vi "Drive Distance to Turn Angle.vi"(5 "Wheelbase (in)":dbl=21.5, 9 "Distance (in)":dbl) -> (3 "Angle (rads)":dbl)   [LabVIEW 2015]
panel:
  # "Arc Length = r * Theta\nTheta = Arc Length / r\nr = 1/2 * wheel base"
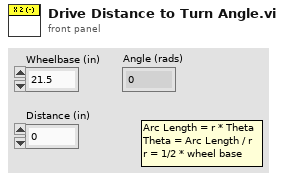
[diagram p1: front panel]
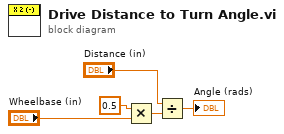
[diagram p0: block diagram]
diagram:
  n1 = Multiply(x=0.5, y="Wheelbase (in)") -> (x*y=w3:dbl)
  n2 = Divide(x="Distance (in)", y=w3) -> (x/y=→"Angle (rads)":dbl)
